vi "AD9910 Check Register Size.vi"(2 "Write Data":u8[](array[numeric]), 3 "Register":T1) -> (0 "# words":i32, 1 "passed":bool)   [LabVIEW 2013, in "DDS.lvlib"]
doc: "Passes if the length of write data is compatible with the given register. # words may give a number greater than 1 if the register is RAM."
uses:
  Controls/AD9910 registers.ctl
  DDS.lvlib
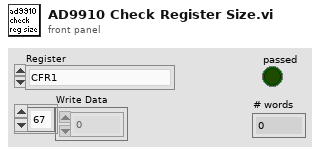
[diagram p1: front panel]
types:
  T1 = typedef "DDS.lvlib/AD9910 registers.ctl" = enum16{"CFR1", "CFR2", "CFR3", "Auxiliary DAC Control", "I/0 Update Rate", "Frequency Tuning Word", "Phase Offset Word", "Amplitude Scale Factor", "Multichip Sync", "Digital Ramp Limit", "Digital Ramp Step Size", "Digital Ramp Rate", "Single Tone Profile 0", "Single Tone Profile 1", "Single Tone Profile 2", "Single Tone Profile 3", "Single Tone Profile 4", "Single Tone Profile 5", "Single Tone Profile 6", "Single Tone Profile 7", "RAM Profile 0", "RAM Profile 1", "RAM Profile 2", "RAM Profile 3", "RAM Profile 4", "RAM Profile 5", "RAM Profile 6", "RAM Profile 7", "RAM"}
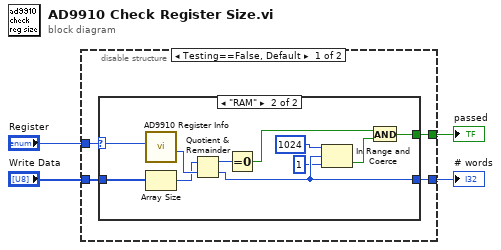
[diagram p0: block diagram]
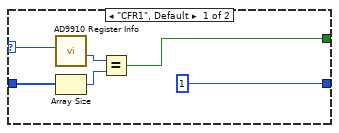
[diagram p2: hidden frame]
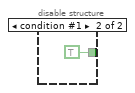
[diagram p3: hidden frame]
diagram:
  n1 = disable-structure shown="Testing==False, Default" {
    disable-tunnel: "Write Data" -> [w8 _]
    disable-tunnel: [w7 TRUE ("passed")] -> w3
    disable-tunnel: "Register" -> [w6 _]
    disable-tunnel: [w5 _] -> w1
    frame condition #0 (active) {
      n2 = case shown="\"RAM\"" w6 {
        selector: w6 -> [w10 w24]
        tunnel: w8 -> [w12 w25]
        tunnel: [w11 w17] -> w7
        tunnel: [1 w20] -> w5
        frame "CFR1", Default {
          n3 = call "AD9910 Register Info.vi"("Register"=w10) -> ("Number of Bytes"=w13:i32)  [unwired: 9 in, 1 out]
          n4 = Array Size(array=w12) -> (size(s)=w14:i32)
          n5 = Equal?(x=w13, y=w14) -> (x = y?=w11:bool)
        }
        frame "RAM" {
          n6 = call "AD9910 Register Info.vi"("Register"=w24) -> ("Number of Bytes"=w23:i32)  [unwired: 9 in, 1 out]
          n7 = Array Size(array=w25) -> (size(s)=w22:i32)
          n8 = Quotient & Remainder(x=w22, y=w23) -> (x-y*floor(x/y)=w21:i32, floor(x/y)=w20:i32)
          n9 = Equal To 0?(x=w21) -> (x = 0?=w15:bool)
          n10 = In Range and Coerce(upper limit=1024, x=w20, lower limit=1) -> (In Range?=w16:bool)  [unwired: 1 out]
          n11 = And(x=w15, y=w16) -> (x .and. y?=w17:bool)
        }
      }
    }
    frame condition #1 {
    }
  }
  "passed" <- w3
  "# words" <- w1
